vi "ControlMotorTest.vi"() -> ()   [LabVIEW 2018]
panel:
  out "数值":i32
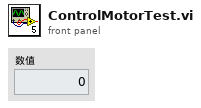
[diagram p1: front panel]
types:
  T1 = typedef "控制电机指令枚举器.ctl" = enum16{"归0", "停止", "运动", "轴设置", "通信连接"}
  T2 = typedef "控制电机位置枚举器.ctl" = enum16{"远场扫描", "发散角扫描", "远场相机", "近场相机", "时间波形", "偏振", "能量", "功率", "光谱"}
  T3 = typedef "控制电机枚举器.ctl" = enum16{"Z", "Y", "X", "发散角", "俯仰", "旋转"}
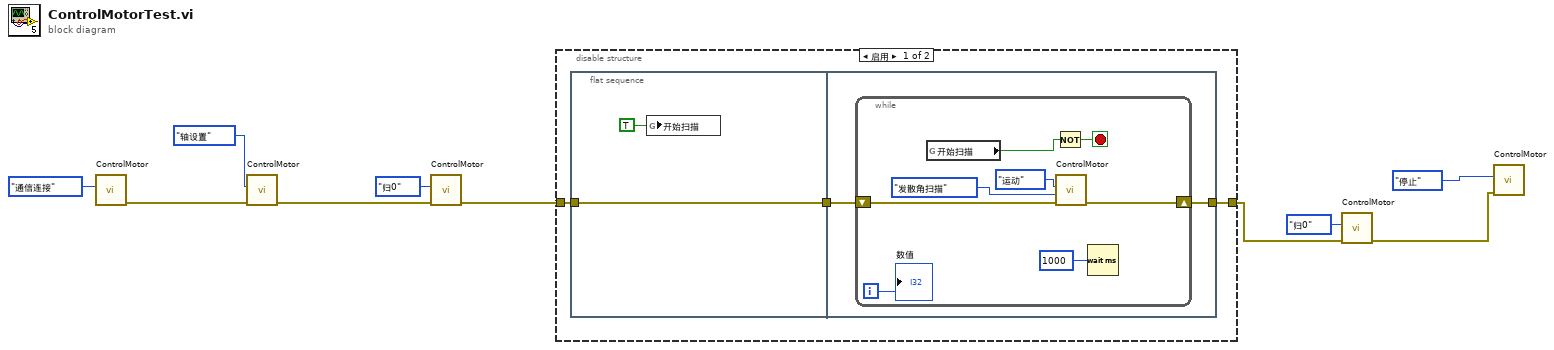
[diagram p0: block diagram]
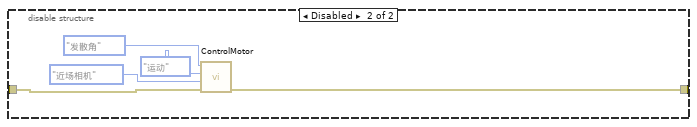
[diagram p2: hidden frame]
diagram:
  n1 = call "ControlMotor.vi"("控制电机指令"=控制电机指令枚举器."通信连接") -> ("错误输出 2"=w9:errorcluster)  [unwired: 7 in]
  n2 = call "ControlMotor.vi"("控制电机指令"=控制电机指令枚举器."轴设置", "错误输入"=w9) -> ("错误输出 2"=w6:errorcluster)  [unwired: 6 in]
  n3 = call "ControlMotor.vi"("控制电机指令"=控制电机指令枚举器."归0", "错误输入"=w6) -> ("错误输出 2"=w5:errorcluster)  [unwired: 6 in]
  n4 = disable-structure shown="启用" {
    disable-tunnel: w5 -> [w13 w30]
    disable-tunnel: [w12 w29] -> w2
    frame Enabled {
      n5 = flat-sequence {
        tunnel: w13 -> [w15]
        tunnel: [w15] -> w11
        tunnel: [w16] -> w12
        tunnel: w11 -> [w17]
        frame #0 {
          n6 = global write "globalMessage.vi" "开始扫描"(TRUE ("开始扫描")) -> ()
        }
        frame #1 {
          n7 = while {
            shift-right: [w22] -> w16
            shift-left: w17 -> [w24]
            i -> [w19]
            stop <- w20 stop-if-true
            n8 = global read "globalMessage.vi" "开始扫描"() -> (w21:bool)
            n9 = Not(x=w21) -> (.not. x?=w20:bool)
            n10 = call "ControlMotor.vi"("控制电机指令"=控制电机指令枚举器."运动", "位置"=控制电机位置枚举器."发散角扫描", "错误输入"=w24) -> ("错误输出 2"=w22:errorcluster)  [unwired: 5 in]
            n11 = Wait (ms)(milliseconds to wait=u32 1000 ("等待时间（毫秒）")) -> ()  [unwired: 1 out]
            "数值" <- w19
          }
        }
      }
    }
    frame Disabled {
      n12 = call "ControlMotor.vi"("错误输入"=w30, "位置"=控制电机位置枚举器."近场相机", "控制电机指令"=控制电机指令枚举器."运动", "控制电机"=控制电机枚举器."发散角") -> ("错误输出 2"=w29:errorcluster)  [unwired: 3 in]
    }
  }
  n13 = call "ControlMotor.vi"("控制电机指令"=控制电机指令枚举器."归0", "错误输入"=w2) -> ("错误输出 2"=w1:errorcluster)  [unwired: 6 in]
  n14 = call "ControlMotor.vi"("控制电机指令"=控制电机指令枚举器."停止", "错误输入"=w1) -> ()  [unwired: 6 in, 1 out]
